vi "Keypad.vi"(8 "error in (no error)":errorcluster, 11 "User_Console_States in":refnum<class "User_Console_States.lvclass">) -> (0 "error out":errorcluster, 3 "State out":refnum<class "State Actor.lvclass">)   [LabVIEW 2025, in "User_Console-ATM.lvlib" / "User_Console_States.lvclass"]
uses:
  User_Console_States.lvclass
  User_Console_States.lvclass/User_Console_States.ctl
  C:/Program Files (x86)/National Instruments/LabVIEW 2025/vi.lib/ni/Actors/State Actor/State Actor/State Actor.lvclass
  C:/Program Files (x86)/National Instruments/LabVIEW 2025/vi.lib/ActorFramework/Actor/Actor.lvclass
  C:/Users/halstead_rideriver/Documents/Labview_Practice/ATM_Machine_Actor Framework/ATM_ACTORFW/User_Console-ATM/User_Console_States/User_Console_States.lvclass
  Keypad/Keypad.lvclass
  C:/Users/halstead_rideriver/Documents/Labview_Practice/ATM_Machine_Actor Framework/ATM_ACTORFW/User_Console-ATM/Keypad/Keypad.lvclass
  <vilib>/ni/Actors/State Actor/State Actor/State Actor.lvclass
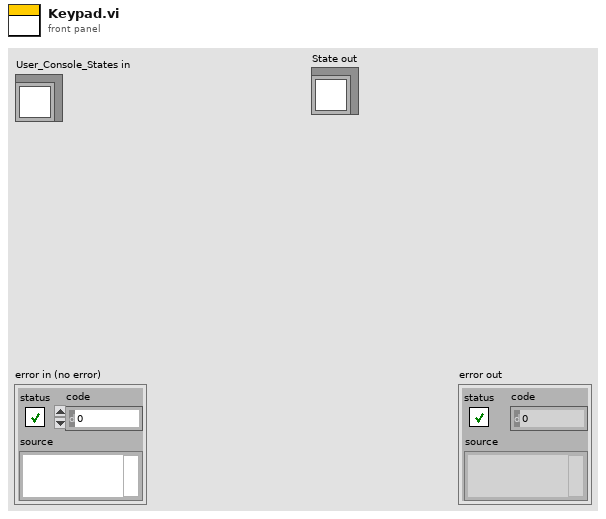
[diagram p1: front panel]
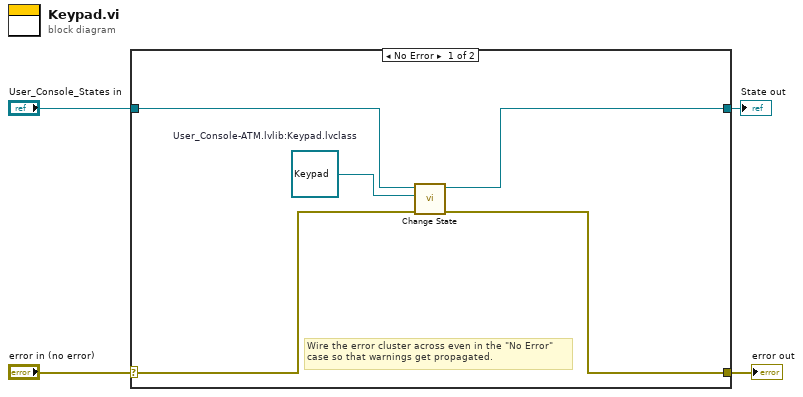
[diagram p0: block diagram]
diagram:
  n1 = case shown="No Error" "error in (no error)" {
    selector: "error in (no error)" -> [w7 w11]
    tunnel: [w6 w11] -> w3
    tunnel: [w8 w10] -> w1
    tunnel: "User_Console_States in" -> [w9 w10]
    frame No Error {
      w5 = refnum<class "Keypad.lvclass"> refnum  # User_Console-ATM.lvlib:Keypad.lvclass
      # "Wire the error cluster across even in the \"No Error\"\ncase so that warnings get propagated."
      n2 = call <vilib>:"Change State.vi"("error in (no error)"=w7, "New State in"=w5, "State in"=w9) -> ("error out"=w6:errorcluster, "State out"=w8:refnum<class "State Actor.lvclass">)  [unwired: 7 in]
    }
    frame Error {
    }
  }
  "error out" <- w3
  "State out" <- w1
